vi "Measurement UI.vi"() -> ()   [LabVIEW 2021, in "PSRR_PMIC_UI.lvlib"]
uses:
  PSRR_PMIC_UI.lvlib
panel:
  in  "MeasGraphs":enum32{"PSRR", "Hidden Controls"}(tab)
  out "PSRRGraph(dB/Hz)":T1(graph)
  in  "Scope resource name":string
  in  "Fgen resource name":string
  out "PSRR":dbl[](array[numeric])
  out "Frequency sweep points":dbl[](array[numeric])
  in  "Load resource name":string
  in  "Source resource name":string caption="RESOURCE NAME"
  in  "MeasConfigurations":T2(tab)
  in  "Load sense":i32(ring)=1009 caption="SENSE" items=["Local"=1008, "Remote"=1009]
  in  "Source sense":i32(ring)=1009 caption="SENSE" items=["Local"=1008, "Remote"=1009]
  in  "DUT setup time":dbl=1.0 caption="DUT SETUP TIME" format="%#_6ps"
  in  "Measurement settings":string="Measurement settings"
  in  "Source configuration":string="Source configuration"
  in  "Load configuration":string="Load configuration"
  in  "Load voltage limit range":dbl=6.0 caption="VOLTAGE LIMIT RANGE" format="%#_6pV"
  in  "Load current level":dbl=0.025 caption="CURRENT LEVEL" format="%#_6pA"
  in  "ELOADResourceName":refnum<k15> caption="RESOURCE NAME"
  in  "Source current limit":dbl=0.15 caption="CURRENT LIMIT" format="%#_6pA"
  in  "Source voltage level":dbl=10.0 caption="VOLTAGE LEVEL" format="%#_6pV"
  in  "PPSResourceName":refnum<k15> caption="RESOURCE NAME"
  in  "Scope output channel name":string caption="OUTPUT CHANNEL NAME"
  in  "Scope cycles to average":i32=4 caption="CYCLES TO AVAERAGE"
  in  "Scope samples per cycle":i32=1000 caption="SAMPLES PER CYCLE"
  in  "Fgen standard Waveform":T3(ring) caption="STANDARD WAVEFORM"
  in  "Fgen sweep type":string(combo)="Logarithmic" caption="SWEEP TYPE"
  in  "Fgen frequency sweep points/points per decade":i32=10 caption="PTS/PTS PER DECADE"
  in  "Fgen stop frequency":dbl=10000000.0 caption="STOP FREQUENCY" format="%#_6pHz"
  in  "Fgen start frequency":dbl=100.0 caption="START FREQUENCY" format="%#_6pHz"
  in  "Fgen load impedance":dbl=10000.0 caption="LOAD IMPEDANCE" format="%#_6pOhm"
  in  "Fgen configuration":string="Fgen configuration"
  in  "Fgen pk-pk amplitude":dbl=1.0 caption="PK-PK AMPLITUDE" format="%#_6pV"
  in  "Fgen channel name":string="0" caption="CHANNEL NAME"
  in  "FGENResourceName":refnum<k15> caption="RESOURCE NAME"
  in  "Scope probe attenuation":dbl=1.0 caption="PROBE ATTENUATION"
  in  "Scope configuration":string="Scope configuration"
  in  "Scope input channel name":string caption="INPUT CHANNEL NAME"
  in  "SCOPEResourceName":refnum<k15> caption="RESOURCE NAME"
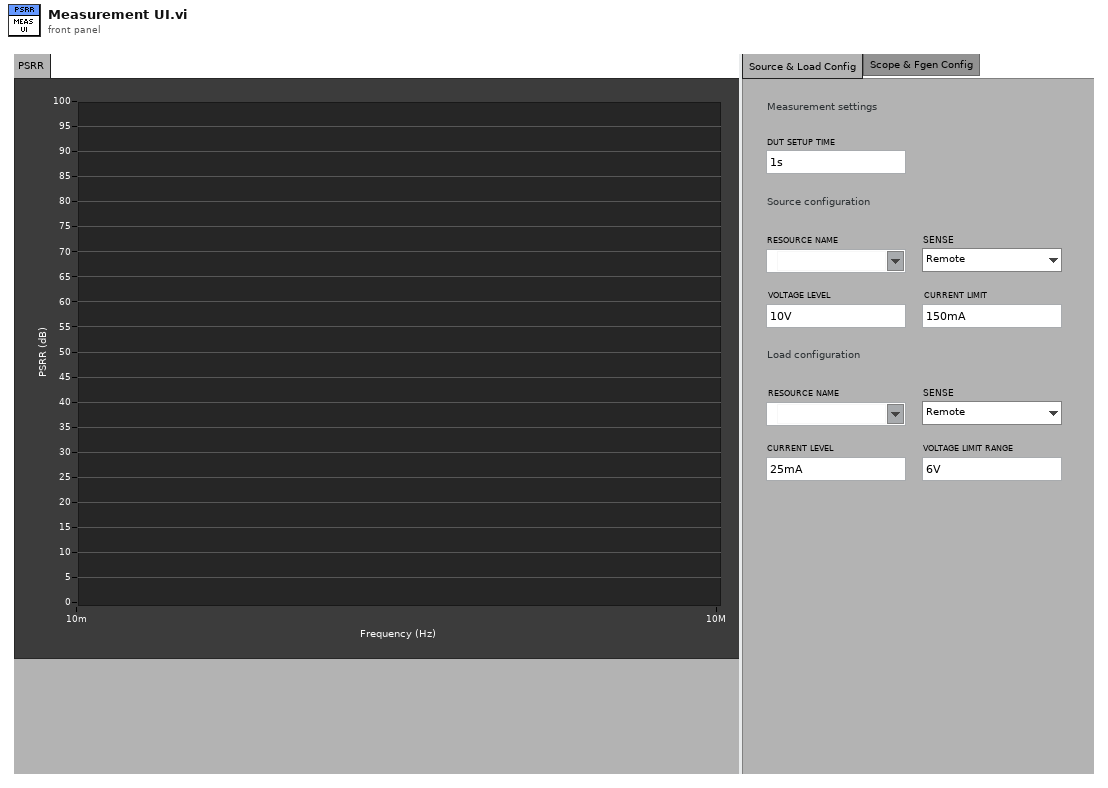
[diagram p1: front panel]
types:
  T1 = cluster{"Source voltages":dbl[], "Load voltages":dbl[]}
  T2 = enum32{"Source & Load Config", "Scope & Fgen Config"}
  T3 = enum32{"Sine", "Square", "Triangle", "Ramp Up", "Ramp Down", "DC", "Noise"}
  T4 = cluster{"Frequency sweep points":dbl[], "PSRR":dbl[]}
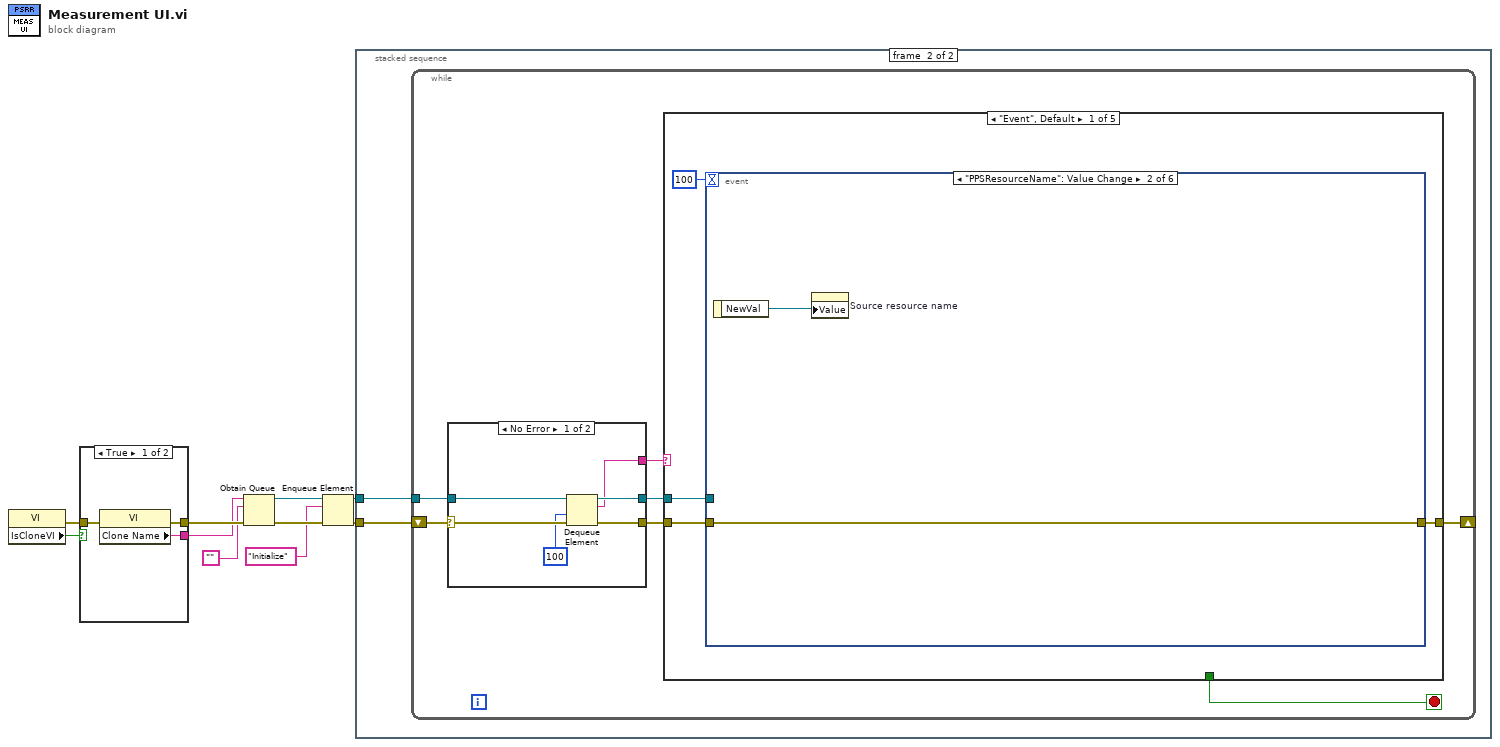
[diagram p0: block diagram]
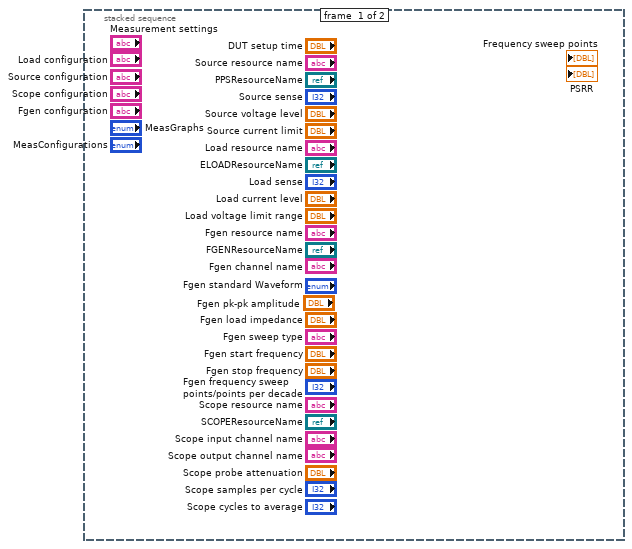
[diagram p2: hidden frame]
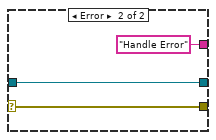
[diagram p3: hidden frame]
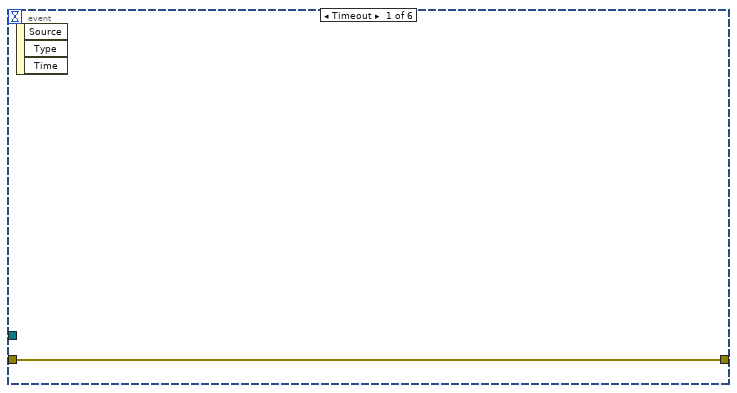
[diagram p4: hidden frame]
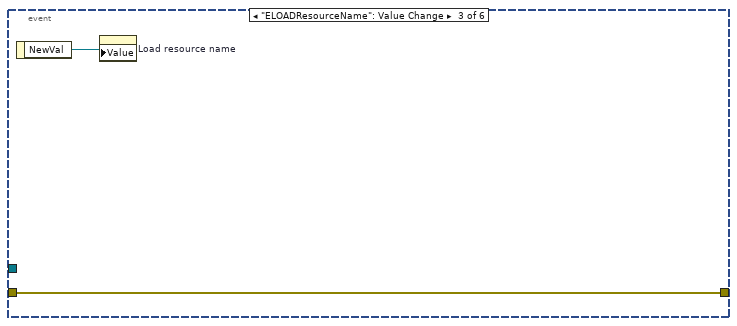
[diagram p5: hidden frame]
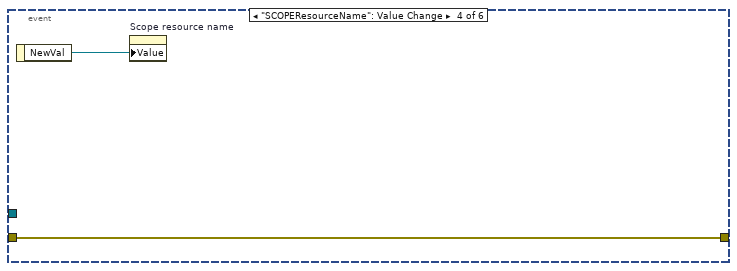
[diagram p6: hidden frame]
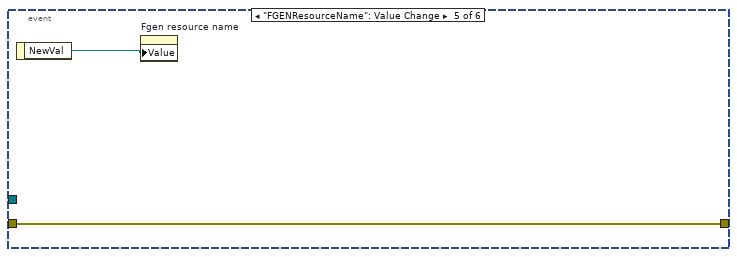
[diagram p7: hidden frame]
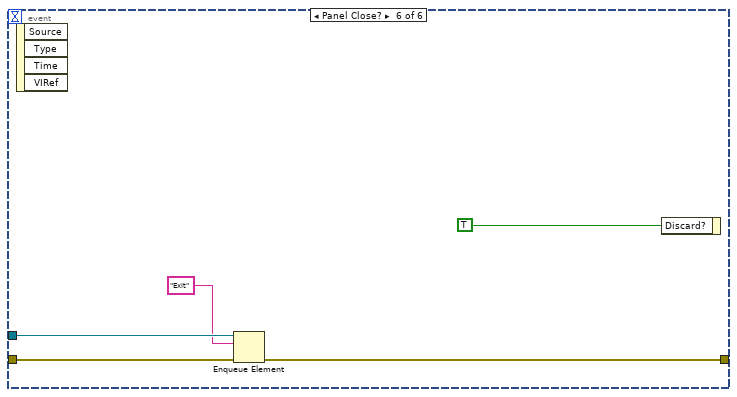
[diagram p8: hidden frame]
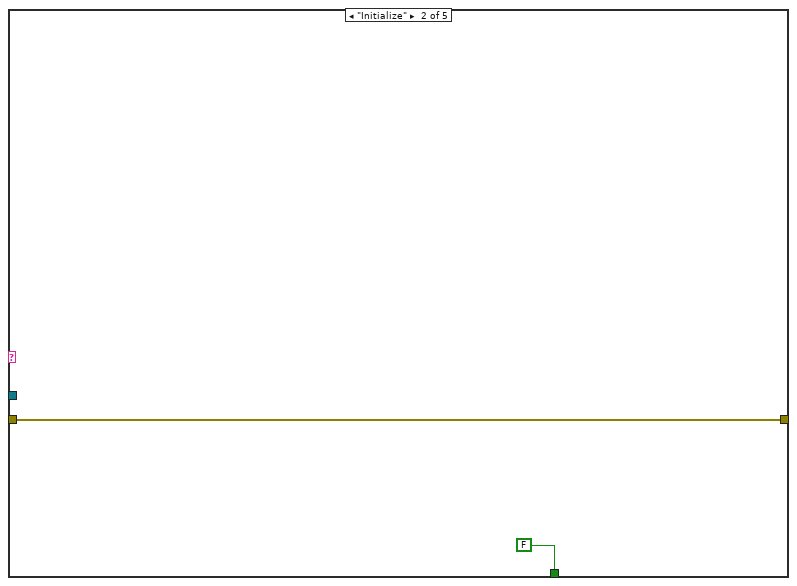
[diagram p9: hidden frame]
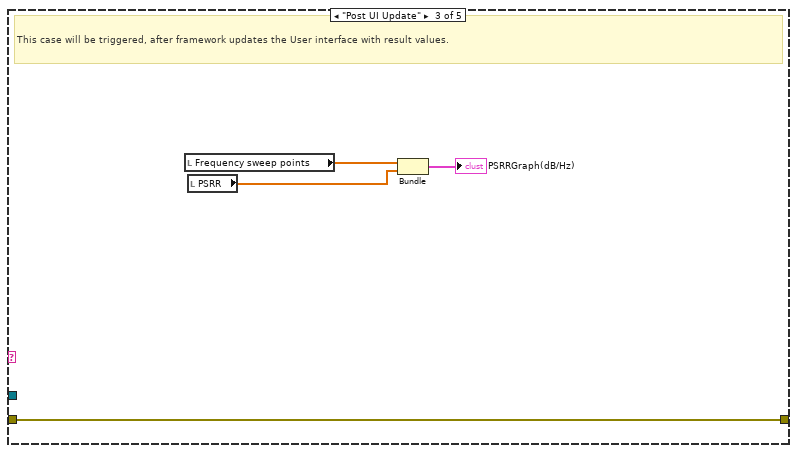
[diagram p10: hidden frame]
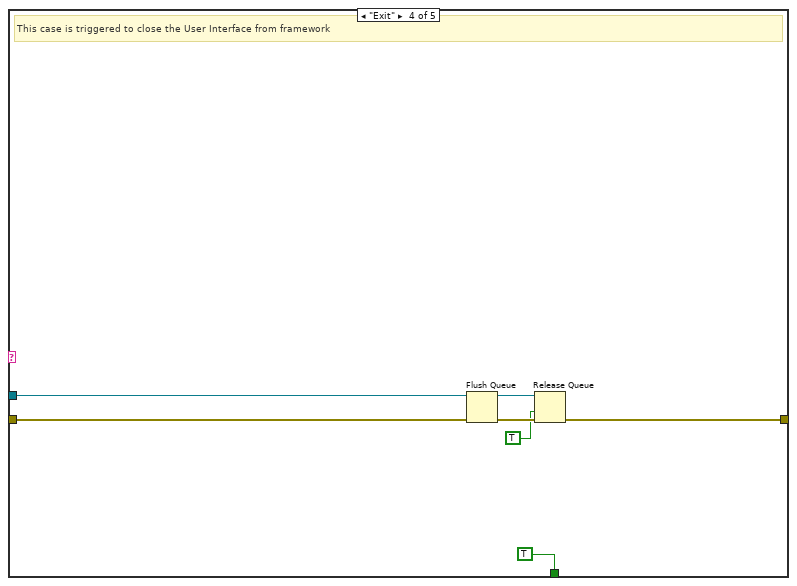
[diagram p11: hidden frame]
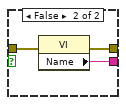
[diagram p13: hidden frame]
diagram:
  n1 = property class="VI"() -> (error out=w1:errorcluster, "IsCloneVI"=w2:bool)  [unwired: 2 in, 1 out]
  n2 = case shown="True" w2 {
    tunnel: [w13 w16] -> w10
    tunnel: [w12 w15] -> w9
    tunnel: w1 -> [w11 w14]
    frame True {
      n3 = property class="VI"(error in=w11) -> (error out=w13:errorcluster, "Clone Name"=w12:string)  [unwired: 1 in, 1 out]
    }
    frame False {
      n4 = property class="VI"(error in=w14) -> (error out=w16:errorcluster, "Name"=w15:string)  [unwired: 1 in, 1 out]
    }
  }
  n5 = Obtain Queue(name (unnamed)=w9, element data type="", error in (no error)=w10) -> (queue out=w6:refnum<queue>, error out=w8:errorcluster)  [unwired: 2 in, 1 out]
  n6 = Enqueue Element(queue=w6, element="Initialize", error in (no error)=w8) -> (queue out=w5:refnum<queue>, error out=w7:errorcluster)  [unwired: 1 in, 1 out]
  n7 = stacked-sequence {
    tunnel: w7 -> [_ w18]
    tunnel: w5 -> [_ w17]
    frame #0 {
    }
    frame #1 {
      n8 = while {
        shift-right: [w20] -> _
        shift-left: w18 -> [w25]
        tunnel: w17 -> [w23]
        stop <- w19 stop-if-true
        n9 = case shown="No Error" w25 {
          selector: w25 -> [w31 w34]
          tunnel: [w30 w34] -> w24
          tunnel: w23 -> [w29 w33]
          tunnel: [w28 w33] -> w22
          tunnel: [w27 "Handle Error"] -> w21
          frame No Error {
            n10 = Dequeue Element(queue=w29, timeout in ms (-1)=100, error in (no error)=w31) -> (queue out=w28:refnum<queue>, element=w27:string, error out=w30:errorcluster)  [unwired: 1 out]
          }
          frame Error {
          }
        }
        n11 = case shown="\"Event\", Default" w21 {
          tunnel: w24 -> [w37 w54 w58 w65 w66]
          tunnel: w22 -> [w35 _ _ w63 _]
          tunnel: [w38 w54 w58 w60 w66] -> w20
          tunnel: [_ FALSE _ TRUE _] -> w19
          frame "Event", Default {
            n12 = event shown="[1] \"PPSResourceName\": Value Change" {
              selector: _ -> [_ _ _ _ _ _]
              dyn-events: _ -> [_ _ _ _ _ _]
              timeout: 100 -> [_ _ _ _ _ _]
              tunnel: [w39 w40 w42 w44 w46 w50] -> w38
              tunnel: w37 -> [w39 w40 w42 w44 w46 w51]
              tunnel: w35 -> [_ _ _ _ _ w49]
              event Timeout {
                n13 = event-data() -> ()  [unwired: 1 in, 3 out]
              }
              event "PPSResourceName": Value Change {
                n14 = event-data() -> ("NewVal"=w41:refnum<k15>)  [unwired: 1 in]
                n15 = property on="Source resource name" class="Str"("Value"=w41) -> ()  [unwired: 2 in, 2 out]
              }
              event "ELOADResourceName": Value Change {
                n16 = event-data() -> ("NewVal"=w43:refnum<k15>)  [unwired: 1 in]
                n17 = property on="Load resource name" class="Str"("Value"=w43) -> ()  [unwired: 2 in, 2 out]
              }
              event "SCOPEResourceName": Value Change {
                n18 = event-data() -> ("NewVal"=w45:refnum<k15>)  [unwired: 1 in]
                n19 = property on="Scope resource name" class="Str"("Value"=w45) -> ()  [unwired: 2 in, 2 out]
              }
              event "FGENResourceName": Value Change {
                n20 = event-data() -> ("NewVal"=w47:refnum<k15>)  [unwired: 1 in]
                n21 = property on="Fgen resource name" class="Str"("Value"=w47) -> ()  [unwired: 2 in, 2 out]
              }
              event Panel Close? {
                n22 = event-data() -> ()  [unwired: 1 in, 4 out]
                n23 = Enqueue Element(queue=w49, element="Exit", error in (no error)=w51) -> (error out=w50:errorcluster)  [unwired: 1 in, 2 out]
                n24 = event-data("Discard?"=TRUE) -> ()  [unwired: 1 in, 1 out]
              }
            }
          }
          frame "Initialize" {
          }
          frame "Post UI Update" {
            # "This case will be triggered, after framework updates the User interface with result values."
            n25 = local read "Frequency sweep points"() -> (w56:dbl[])
            n26 = local read "PSRR"() -> (w55:dbl[])
            n27 = Bundle("Frequency sweep points"=w56, "PSRR"=w55) -> (→"PSRRGraph(dB/Hz)":T4)  [unwired: 1 in]
          }
          frame "Exit" {
            # "This case is triggered to close the User Interface from framework"
            n28 = Flush Queue(queue=w63, error in (no error)=w65) -> (queue out=w62:refnum<queue>, error out=w61:errorcluster)  [unwired: 1 out]
            n29 = Release Queue(queue=w62, force destroy? (F)=TRUE, error in (no error)=w61) -> (error out=w60:errorcluster)  [unwired: 2 out]
          }
          frame "Handle Error" {
          }
        }
      }
    }
  }
